vi "Clocked Output.vi"() -> ()   [LabVIEW 2021]
doc: "This example demonstrates how to generate a finite amount of data from a buffer in your computer's memory."
uses:
  <vilib>/Utility/error.llb/DialogType.ctl
  <vilib>/DAQmx/write.llb/DAQmx Write (Analog 1D DBL 1Chan NSamp).vi
  <vilib>/DAQmx/create/channels.llb/DAQmx Create Channel (AO-Voltage-Basic).vi
  <vilib>/DAQmx/configure/timing.llb/DAQmx Timing (Sample Clock).vi
  <vilib>/DAQmx/miscellaneous.llb/DAQmx Fill In Error Info.vi
  <resource>/objmgr/daqmx.rc
panel:
  in  "stop":bool
  in  "Send":bool
  out "Waveform Graph":dbl[][](graph)
  in  "Physical Channel(s)":tag="Dev2/ao0"
  out "Actual Sample Rate":dbl=1000.0 format="%0.2f"
  # "Channel Settings"
  # "Output"
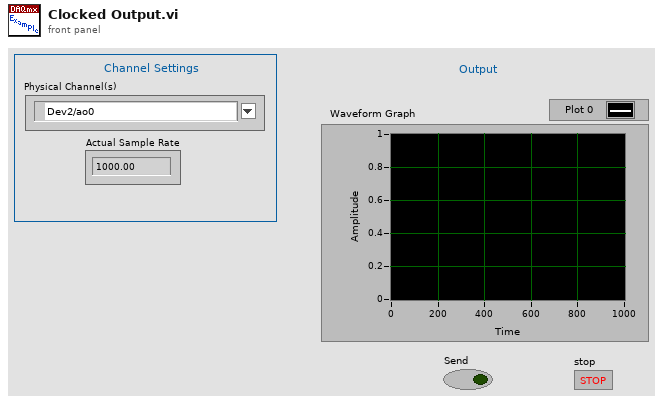
[diagram p1: front panel]
types:
  T1 = typedef "DialogType.ctl" = u16
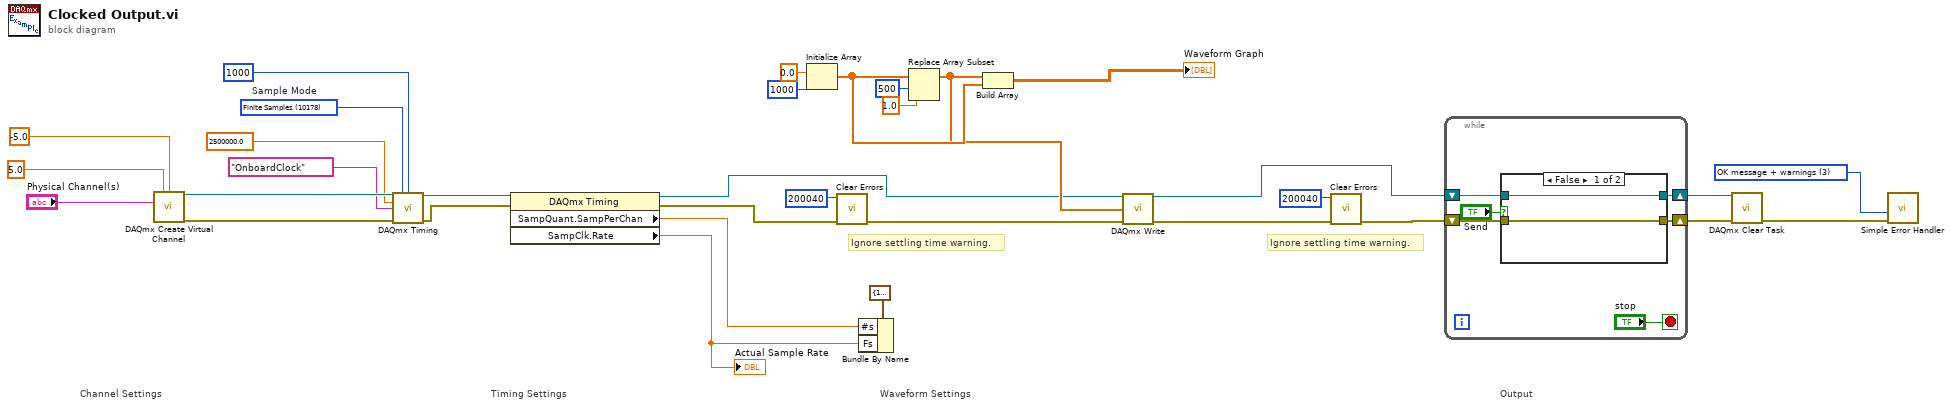
[diagram p0: block diagram]
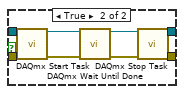
[diagram p2: hidden frame]
diagram:
  w16 = T1 3 items=["no dialog", "OK message", "continue or stop message", "OK message + warnings", "continue/stop + warnings"] ("type of dialog (OK msg:1)")
  w31 = 10178 items=["Finite Samples"=10178, "Continuous Samples"=10123, "Hardware Timed Single Point"=12522]  # Sample Mode
  # "Ignore settling time warning."
  # "Ignore settling time warning."
  # "Output"
  # "Waveform Settings"
  # "Timing Settings"
  # "Channel Settings"
  n1 = call-poly <vilib>:"DAQmx Create Virtual Channel.vi"("maximum value"=5.0 ("Max Voltage"), "minimum value"=-5.0 ("Min Voltage"), "physical channels"="Physical Channel(s)") -> ("task out"=w29:refnum<k21>, "error out"=w30:errorcluster)  [unwired: 11 in]
  n2 = call-poly <vilib>:"DAQmx Timing.vi"("task/channels in"=w29, "sample mode"=w31, "samples per channel"=1000 ("Number of Samples"), "rate"=2500000.0 ("Sample Rate"), "source"=tag "OnboardClock" ("Sample Clock Source"), "error in"=w30) -> ("task out"=w33:refnum<k21>, "error out"=w32:errorcluster)  [unwired: 8 in]
  n3 = property class="DAQmx Timing"(reference=w33, error in=w32) -> (reference out=w5:refnum<k21>, error out=w15:errorcluster, "SampQuant.SampPerChan"=w20:dbl, "SampClk.Rate"=w19:dbl)
  "Actual Sample Rate" <- w19
  n4 = Initialize Array(0.0 ("element"), 1000 ("dimension size")) -> (w10:dbl[])
  n5 = call <vilib>:"Clear Errors.vi"("error in (no error)"=w15, "specific error code to clear (0: all)"=200040) -> ("error out"=w7:errorcluster)  [unwired: 4 in, 1 out]
  n6 = Bundle By Name(cluster=cluster{"Fs":dbl, "#s":dbl} {"Fs"=1000.0, "#s"=1000.0} ("sampling info"), "#s"=w20, "Fs"=w19) -> ()  [unwired: 1 out]
  n7 = Replace Array Subset(array=w10, new element=1.0 ("new element/subarray"), index=500) -> (w9:dbl[])
  n8 = Build Array(w9, w10) -> (→"Waveform Graph":dbl[][])
  n9 = call-poly <vilib>:"DAQmx Write.vi"("task/channels in"=w5, "data"=w9, "error in"=w7) -> ("task out"=w1:refnum<k21>, "error out"=w3:errorcluster)  [unwired: 10 in, 1 out]
  n10 = call <vilib>:"Clear Errors.vi"("error in (no error)"=w3, "specific error code to clear (0: all)"=200040) -> ("error out"=w2:errorcluster)  [unwired: 4 in, 1 out]
  n11 = while {
    shift-right: [w38] -> w17
    shift-left: w2 -> [w37]
    shift-right: [w39] -> w18
    shift-left: w1 -> [w36]
    stop <- "stop" stop-if-true
    n12 = case shown="False" "Send" {
      tunnel: [w40 w47] -> w39
      tunnel: [w41 w46] -> w38
      tunnel: w37 -> [w41 w43]
      tunnel: w36 -> [w40 w42]
      frame False {
      }
      frame True {
        n13 = call <vilib>:"DAQmx Start Task.vi"("task/channels in"=w42, "error in"=w43) -> ("task out"=w49:refnum<k21>, "error out"=w48:errorcluster)  [unwired: 12 in]
        n14 = call <vilib>:"DAQmx Wait Until Done.vi"("task/channels in"=w49, "error in"=w48) -> ("task out"=w45:refnum<k21>, "error out"=w44:errorcluster)  [unwired: 12 in]
        n15 = call <vilib>:"DAQmx Stop Task.vi"("task/channels in"=w45, "error in"=w44) -> ("task out"=w47:refnum<k21>, "error out"=w46:errorcluster)  [unwired: 12 in]
      }
    }
  }
  n16 = call <vilib>:"DAQmx Clear Task.vi"("task in"=w18, "error in"=w17) -> ("error out"=w28:errorcluster)  [unwired: 13 in]
  n17 = call <vilib>:"Simple Error Handler.vi"("type of dialog (OK msg:1)"=w16, "error in (no error)"=w28) -> ()  [unwired: 3 in, 5 out]
